vi "reheat.vi"(8 "error in (no error)":errorcluster, 11 "Microwave in":refnum<class "Microwave.lvclass">) -> (0 "error out":errorcluster, 3 "Microwave out":refnum<class "Microwave.lvclass">)   [LabVIEW 2010, in "Microwave.lvclass"]
uses:
  Microwave.lvclass
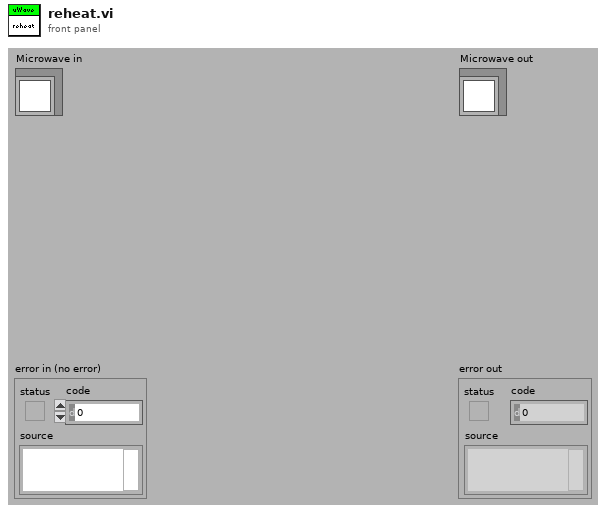
[diagram p1: front panel]
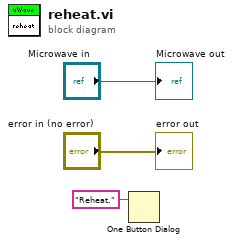
[diagram p0: block diagram]
diagram:
  n1 = One Button Dialog(message="Reheat.") -> ()  [unwired: 1 in, 1 out]
  "error out" <- "error in (no error)"
  "Microwave out" <- "Microwave in"
